vi "Configure Detector Mode.vi"(8 "error in (no error)":errorcluster, 10 "Detector Mode":T1(ring), 11 "SA-FSW in":refnum<class "SA-FSW.lvclass">) -> (0 "error out":errorcluster, 3 "SA-FSW out":refnum<class "SA-FSW.lvclass">)   [LabVIEW 2020, in "SA-FSW.lvclass"]
uses:
  SA-FSW.lvclass
  C:/Sandbox/RF Bench/Source Code/WiSpry Test Framework/Instruments/Spectrum Analyzer/Spectrum Analyzer.lvclass
  C:/Sandbox/RF Bench/Source Code/WiSpry Test Framework/Instruments/Instrument.lvclass
  Instrument.lvclass/Instrument.ctl
  Spectrum Analyzer.lvclass/Spectrum Analyzer.ctl
  Spectrum Analyzer.lvclass
  Instrument.lvclass
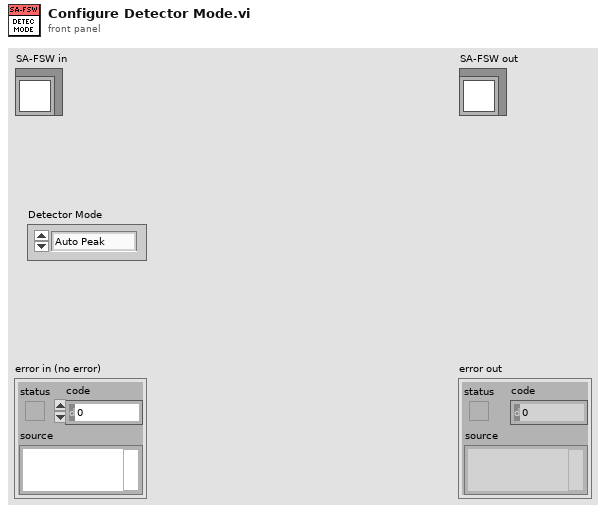
[diagram p1: front panel]
types:
  T1 = enum16{"Auto Peak", "Negative Peak", "Positive Peak", "Quasipeak", "Sample", "RMS", "Average", "CISPR Average", "CISPR RMS"}
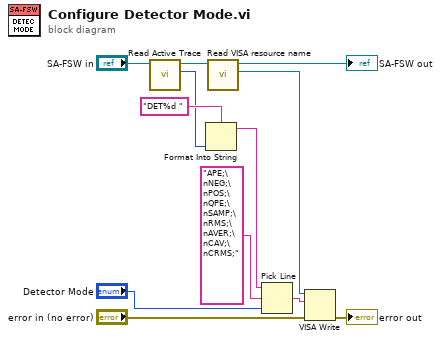
[diagram p0: block diagram]
diagram:
  n1 = call "Read Active Trace.vi"("Spectrum Analyzer in"="SA-FSW in") -> ("Active Trace"=w10:u16, "Spectrum Analyzer out"=w6:refnum<class "SA-FSW.lvclass">)  [unwired: 9 in]
  n2 = Format Into String(format string="DET%d " ("string (\"\")"), w10) -> (resulting string=w9:string)  [unwired: 2 in, 1 out]
  n3 = call "Read VISA resource name.vi"("Instrument in"=w6) -> ("VISA resource name"=w5:refnum<visa-resource-name>, "Instrument out"=→"SA-FSW out":refnum<class "SA-FSW.lvclass">)  [unwired: 9 in]
  n4 = Pick Line(string ("")=w9, multi-line string="APE;\nNEG;\nPOS;\nQPE;\nSAMP;\nRMS;\nAVER;\nCAV;\nCRMS;", line index="Detector Mode") -> (output string=w3:string)
  n5 = VISA Write(VISA resource name=w5, write buffer=w3, error in (no error)="error in (no error)") -> (error out=→"error out":errorcluster)  [unwired: 2 out]
